vi "Motor_inlt.vi"(8 "에러 입력(에러 없음)":errorcluster) -> (0 "에러 출력":errorcluster)   [LabVIEW 2019]
uses:
  <vilib>/Platform/TimedLoop/XDataNode/timing_clust.ctl
  <vilib>/Platform/TimedLoop/XDataNode/nitl_modes.ctl
  <vilib>/Platform/TimedLoop/XDataNode/wakeup.ctl
  Type/SDO_Command.ctl
  <vilib>/Platform/TimedLoop/XDataNode/XDataNode.xnode
  <vilib>/Platform/TimedLoop/XDataNode/XDNodeRunTimeDep.lvlib
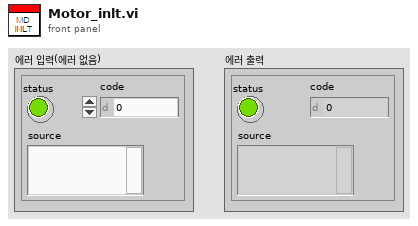
[diagram p1: front panel]
types:
  T1 = typedef "XDNodeRunTimeDep.lvlib/timing_clust.ctl" = cluster{"Expected End [f-1]":u64, "Actual End [f-1]":u64, "Finished Late? [f-1]":bool, "Expected End [i-1]":u64, "Actual End [i-1]":u64, "Finished Late? [i-1]":bool, "Expected Start [i]":u64, "Actual Start [i]":u64, "Expected Start [f]":u64, "Actual Start [f]":u64, "Source Name":string, "Structure Name":string, "Period":i64, "Deadline":i64, "Offset":i64, "Start":i64, "Priority":i32, "Timeout":i32, "Mode":T2, "Wakeup Reason":T3, "Error":errorcluster, "Source Type":string, "Secondary Source Type":string, "Global End Time":u64, "Global Start Time":u64, "Frame Duration":u64, "Iteration Duration":u64, "Assigned CPU":i32, "I/O Scan Engine Mode":u32}
  T2 = typedef "XDNodeRunTimeDep.lvlib/nitl_modes.ctl" = enum32{"No Change", "Process missed periods, maintain original phase", "Discard missed periods, maintain original phase", "Process missed periods, ignore original phase", "Discard missed periods, ignore original phase"}
  T3 = typedef "XDNodeRunTimeDep.lvlib/wakeup.ctl" = enum32{"Normal", "Aborted", "Asynchronous wakeup", "Timing source error", "Timed loop error", "Timeout"}
  T4 = cluster{"Target":i32, "Manual":u8[], "Velocity":u32, "Acc/Dec":u32}
  T5 = typedef "SDO_Command.ctl" = enum16{"Idle", "Shutdown", "Switch On", "Enable Operation", "Disable Voltage", "Quikstop", "Disable Operation", "Fault Reset", "Manual", "Statusword", "Mode of Operation", "Mode Display", "Target Position", "Position Actual Value", "Controlword_Move", "Profile Velocity", "Profile Acceleration", "Profile Deceleration", "Move"}
  T6 = typedef "CANFrameControl.ctl" = cluster{"identifier":u32, "extended?":bool, "type":u8, "payload":u8[]}
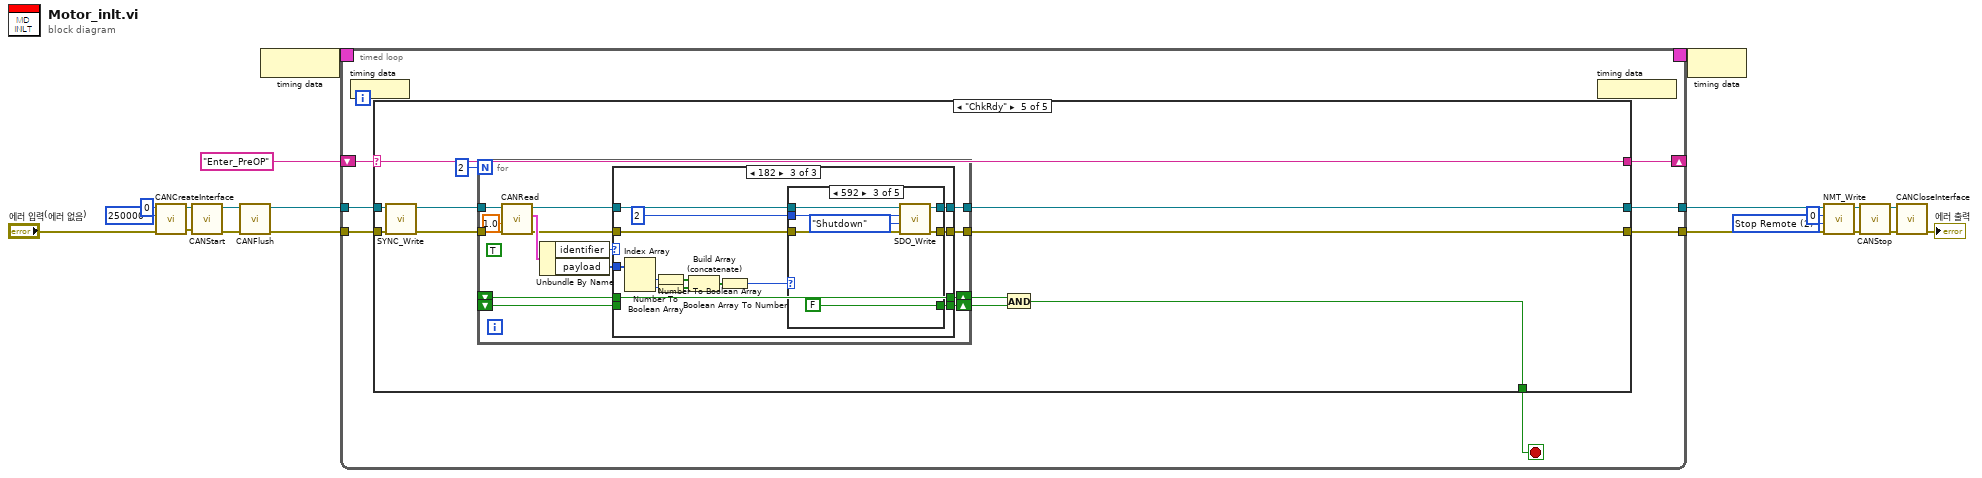
[diagram p0: block diagram]
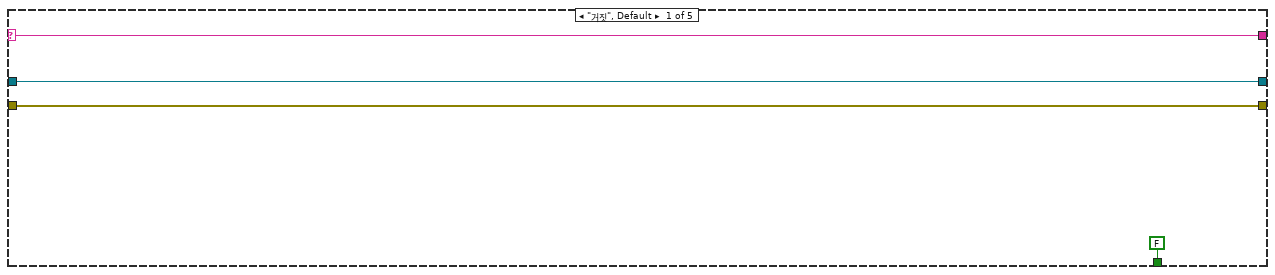
[diagram p2: hidden frame]
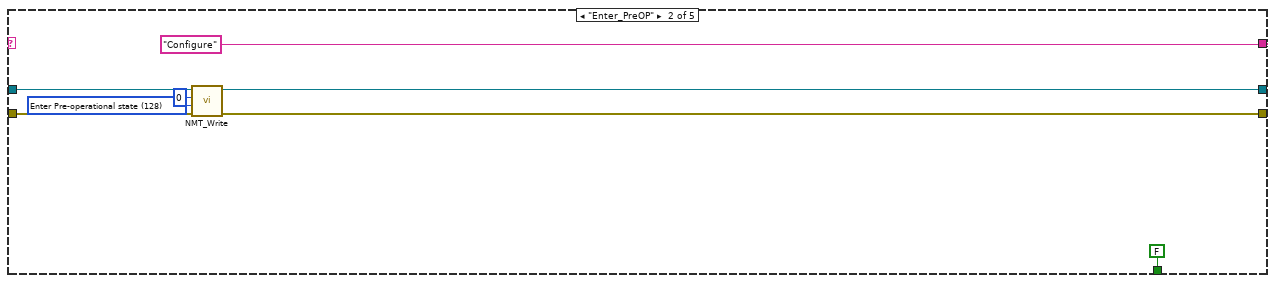
[diagram p3: hidden frame]
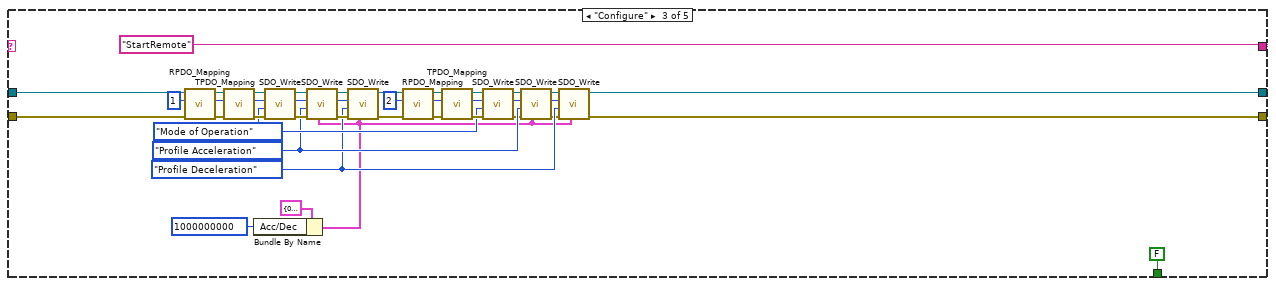
[diagram p4: hidden frame]
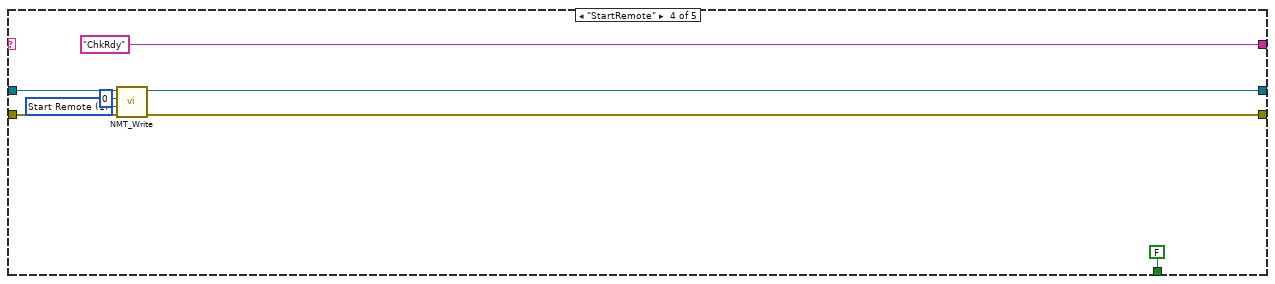
[diagram p5: hidden frame]
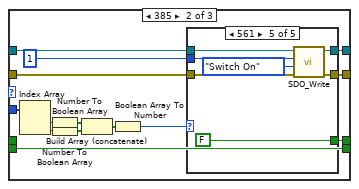
[diagram p7: hidden frame]
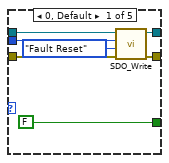
[diagram p8: hidden frame]
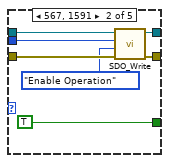
[diagram p9: hidden frame]
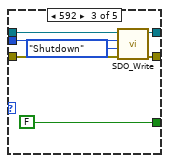
[diagram p10: hidden frame]
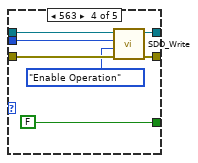
[diagram p11: hidden frame]
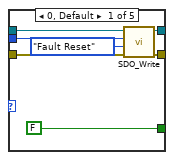
[diagram p12: hidden frame]
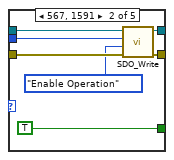
[diagram p13: hidden frame]
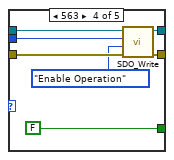
[diagram p14: hidden frame]
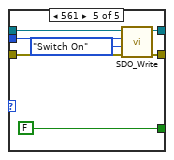
[diagram p15: hidden frame]
diagram:
  w15 = u8 2 items=["Start Remote"=1, "Stop Remote"=2, "Enter Pre-operational state"=128, "Reset node"=129, "Reset communication"=130] ("Command")
  n1 = call <vilib>:"CANCreateInterface.vi"("error in (no error)"="에러 입력(에러 없음)", "baud rate (125000 bps)"=u32 250000, "interface index"=u32 0) -> ("error out"=w4:errorcluster, "interface object out"=w3:refnum<k20>)  [unwired: 7 in]
  n2 = call <vilib>:"CANStart.vi"("error in (no error)"=w4, "interface object in"=w3) -> ("error out"=w7:errorcluster, "interface object out"=w6:refnum<k20>)  [unwired: 8 in]
  n3 = call <vilib>:"CANFlush.vi"("error in (no error)"=w7, "interface object in"=w6) -> ("error out"=w9:errorcluster, "interface object out"=w8:refnum<k20>)  [unwired: 8 in]
  n4 = node-c288() -> (w21:T1)
  n5 = timed-loop {
    shift-right: [w28] -> _
    shift-left: "Enter_PreOP" -> [w27]
    tunnel: [w26] -> w17
    timing: w21 -> [_]
    timing-out: [_] -> w20
    tunnel: w9 -> [w24]
    tunnel: w8 -> [w23]
    tunnel: [w25] -> w16
    stop <- w22 stop-if-true
    n6 = node-c288() -> ()  [unwired: 1 in]
    n7 = case shown="\"ChkRdy\"" w27 {
      selector: w27 -> [w34 _ _ _ w84]
      tunnel: [w34 "Configure" "StartRemote" "ChkRdy" w84] -> w28
      tunnel: [w33 w37 w45 w77 w89] -> w25
      tunnel: w23 -> [w33 w40 w48 w80 w91]
      tunnel: [w32 w36 w44 w76 w88] -> w26
      tunnel: w24 -> [w32 w39 w47 w79 w90]
      tunnel: [FALSE FALSE FALSE FALSE w83] -> w22
      frame "거짓", Default {
      }
      frame "Enter_PreOP" {
        w42 = u8 128 items=["Start Remote"=1, "Stop Remote"=2, "Enter Pre-operational state"=128, "Reset node"=129, "Reset communication"=130] ("Command")
        n8 = call "NMT_Write.vi"("error in"=w39, "Command"=w42, "Node_ID"=u32 0, "interface object in"=w40) -> ("error out"=w36:errorcluster, "interface object out"=w37:refnum<k20>)  [unwired: 6 in]
      }
      frame "Configure" {
        w52 = SDO_Command."Profile Deceleration" ("Command")
        w53 = SDO_Command."Profile Acceleration" ("Command")
        w54 = u32 2 ("Node_ID")
        w65 = u32 1 ("Node_ID")
        w57 = SDO_Command."Mode of Operation" ("Command")
        n9 = call "RPDO_Mapping.vi"("error in"=w47, "Node_ID"=w65, "interface object in"=w48) -> ("error out"=w73:errorcluster, "interface object out"=w74:refnum<k20>)  [unwired: 7 in]
        n10 = call "TPDO_Mapping.vi"("error in"=w73, "Node_ID"=w65, "interface object in"=w74) -> ("error out"=w71:errorcluster, "interface object out"=w72:refnum<k20>)  [unwired: 7 in]
        n11 = Bundle By Name(cluster=T4 {"Target"=0, "Manual"=[], "Velocity"=0, "Acc/Dec"=0} ("Parameter"), "Acc/Dec"=u32 1000000000) -> (w51:T4)
        n12 = call "SDO_Write.vi"("error in"=w71, "Command"=w57, "Node_ID"=w65, "interface object in"=w72) -> ("error out"=w64:errorcluster, "interface object out"=w63:refnum<k20>)  [unwired: 6 in]
        n13 = call "SDO_Write.vi"("Parameter"=w51, "error in"=w64, "Command"=w53, "Node_ID"=w65, "interface object in"=w63) -> ("error out"=w62:errorcluster, "interface object out"=w66:refnum<k20>)  [unwired: 5 in]
        n14 = call "SDO_Write.vi"("Parameter"=w51, "error in"=w62, "Command"=w52, "Node_ID"=w65, "interface object in"=w66) -> ("error out"=w58:errorcluster, "interface object out"=w59:refnum<k20>)  [unwired: 5 in]
        n15 = call "RPDO_Mapping.vi"("error in"=w58, "Node_ID"=w54, "interface object in"=w59) -> ("error out"=w69:errorcluster, "interface object out"=w70:refnum<k20>)  [unwired: 7 in]
        n16 = call "TPDO_Mapping.vi"("error in"=w69, "Node_ID"=w54, "interface object in"=w70) -> ("error out"=w67:errorcluster, "interface object out"=w68:refnum<k20>)  [unwired: 7 in]
        n17 = call "SDO_Write.vi"("error in"=w67, "Command"=w57, "Node_ID"=w54, "interface object in"=w68) -> ("error out"=w50:errorcluster, "interface object out"=w56:refnum<k20>)  [unwired: 6 in]
        n18 = call "SDO_Write.vi"("Parameter"=w51, "error in"=w50, "Command"=w53, "Node_ID"=w54, "interface object in"=w56) -> ("error out"=w49:errorcluster, "interface object out"=w55:refnum<k20>)  [unwired: 5 in]
        n19 = call "SDO_Write.vi"("Parameter"=w51, "error in"=w49, "Command"=w52, "Node_ID"=w54, "interface object in"=w55) -> ("error out"=w44:errorcluster, "interface object out"=w45:refnum<k20>)  [unwired: 5 in]
      }
      frame "StartRemote" {
        w81 = u8 1 items=["Start Remote"=1, "Stop Remote"=2, "Enter Pre-operational state"=128, "Reset node"=129, "Reset communication"=130] ("Command")
        n20 = call "NMT_Write.vi"("error in"=w79, "Command"=w81, "Node_ID"=u32 0, "interface object in"=w80) -> ("error out"=w76:errorcluster, "interface object out"=w77:refnum<k20>)  [unwired: 6 in]
      }
      frame "ChkRdy" {
        n21 = call "SYNC_Write.vi"("error in"=w90, "interface object in"=w91) -> ("error out"=w92:errorcluster, "interface object out"=w93:refnum<k20>)  [unwired: 8 in]
        n22 = for {
          N: 2 -> [_]
          tunnel: w93 -> [w102]
          tunnel: [w99] -> w89
          tunnel: w92 -> [w101]
          tunnel: [w98] -> w88
          shift-right: [w97] -> w87
          shift-left: _ -> [w95]
          shift-right: [w96] -> w86
          shift-left: _ -> [w94]
          (unwired) TRUE
          n23 = call <vilib>:"CANRead.vi"("error in (no error)"=w101, "timeout (0 s)"=1.0, "interface object in"=w102) -> ("error out"=w103:errorcluster, "CAN frame"=w107:T6, "interface object out"=w104:refnum<k20>)  [unwired: 5 in, 1 out]
          n24 = Unbundle By Name(w107) -> ("identifier"=w106:u32, "payload"=w105:u8[])
          n25 = case shown="182" w106 {
            tunnel: w105 -> [_ w120 w169]
            tunnel: w104 -> [w110 w119 w166]
            tunnel: w103 -> [w111 w118 w165]
            tunnel: [w111 w117 w167] -> w98
            tunnel: [w110 w116 w168] -> w99
            tunnel: [w109 w114 w161] -> w97
            tunnel: [w108 w112 w163] -> w96
            tunnel: w95 -> [w109 _ w161]
            tunnel: w94 -> [w108 w112 _]
            frame 0, Default {
            }
            frame 385 {
              n26 = Index Array(array=w120) -> (element #1=w125:u8, element #2=w124:u8)  [unwired: 2 in]
              n27 = Number To Boolean Array(number=w125) -> (Boolean array=w123:bool[])
              n28 = Number To Boolean Array(number=w124) -> (Boolean array=w122:bool[])
              n29 = Build Array (concatenate)(w123, w122) -> (w121:bool[])
              n30 = Boolean Array To Number(Boolean array=w121) -> (number=w115:u32)
              n31 = case shown="561" w115 {
                tunnel: u32 1 -> [w130 w137 w144 w151 w158]
                tunnel: w119 -> [w131 w138 w145 w150 w159]
                tunnel: w118 -> [w129 w136 w143 w152 w157]
                tunnel: [FALSE TRUE FALSE FALSE FALSE] -> w114
                tunnel: [w127 w135 w141 w149 w156] -> w116
                tunnel: [w128 w134 w142 w148 w155] -> w117
                frame 0, Default {
                  n32 = call "SDO_Write.vi"("error in"=w129, "Command"=SDO_Command."Fault Reset", "Node_ID"=w130, "interface object in"=w131) -> ("error out"=w128:errorcluster, "interface object out"=w127:refnum<k20>)  [unwired: 6 in]
                }
                frame 567, 1591 {
                  n33 = call "SDO_Write.vi"("error in"=w136, "Command"=SDO_Command."Enable Operation", "Node_ID"=w137, "interface object in"=w138) -> ("error out"=w134:errorcluster, "interface object out"=w135:refnum<k20>)  [unwired: 6 in]
                }
                frame 592 {
                  n34 = call "SDO_Write.vi"("error in"=w143, "Command"=SDO_Command."Shutdown", "Node_ID"=w144, "interface object in"=w145) -> ("error out"=w142:errorcluster, "interface object out"=w141:refnum<k20>)  [unwired: 6 in]
                }
                frame 563 {
                  n35 = call "SDO_Write.vi"("error in"=w152, "Command"=SDO_Command."Enable Operation", "Node_ID"=w151, "interface object in"=w150) -> ("error out"=w148:errorcluster, "interface object out"=w149:refnum<k20>)  [unwired: 6 in]
                }
                frame 561 {
                  n36 = call "SDO_Write.vi"("error in"=w157, "Command"=SDO_Command."Switch On", "Node_ID"=w158, "interface object in"=w159) -> ("error out"=w155:errorcluster, "interface object out"=w156:refnum<k20>)  [unwired: 6 in]
                }
              }
            }
            frame 386 {
              n37 = Index Array(array=w169) -> (element #1=w174:u8, element #2=w173:u8)  [unwired: 2 in]
              n38 = Number To Boolean Array(number=w174) -> (Boolean array=w172:bool[])
              n39 = Number To Boolean Array(number=w173) -> (Boolean array=w171:bool[])
              n40 = Build Array (concatenate)(w172, w171) -> (w170:bool[])
              n41 = Boolean Array To Number(Boolean array=w170) -> (number=w164:u32)
              n42 = case shown="592" w164 {
                tunnel: u32 2 -> [w179 w185 w193 w200 w207]
                tunnel: w166 -> [w180 w186 w194 w201 w208]
                tunnel: w165 -> [w178 w187 w192 w199 w206]
                tunnel: [FALSE TRUE FALSE FALSE FALSE] -> w163
                tunnel: [w177 w184 w191 w198 w205] -> w168
                tunnel: [w176 w183 w190 w197 w204] -> w167
                frame 0, Default {
                  n43 = call "SDO_Write.vi"("error in"=w178, "Command"=SDO_Command."Fault Reset", "Node_ID"=w179, "interface object in"=w180) -> ("error out"=w176:errorcluster, "interface object out"=w177:refnum<k20>)  [unwired: 6 in]
                }
                frame 567, 1591 {
                  n44 = call "SDO_Write.vi"("error in"=w187, "Command"=SDO_Command."Enable Operation", "Node_ID"=w185, "interface object in"=w186) -> ("error out"=w183:errorcluster, "interface object out"=w184:refnum<k20>)  [unwired: 6 in]
                }
                frame 592 {
                  n45 = call "SDO_Write.vi"("error in"=w192, "Command"=SDO_Command."Shutdown", "Node_ID"=w193, "interface object in"=w194) -> ("error out"=w190:errorcluster, "interface object out"=w191:refnum<k20>)  [unwired: 6 in]
                }
                frame 563 {
                  n46 = call "SDO_Write.vi"("error in"=w199, "Command"=SDO_Command."Enable Operation", "Node_ID"=w200, "interface object in"=w201) -> ("error out"=w197:errorcluster, "interface object out"=w198:refnum<k20>)  [unwired: 6 in]
                }
                frame 561 {
                  n47 = call "SDO_Write.vi"("error in"=w206, "Command"=SDO_Command."Switch On", "Node_ID"=w207, "interface object in"=w208) -> ("error out"=w204:errorcluster, "interface object out"=w205:refnum<k20>)  [unwired: 6 in]
                }
              }
            }
          }
        }
        n48 = And(x=w87, y=w86) -> (x .and. y?=w83:bool)
      }
    }
    n49 = node-c288() -> ()  [unwired: 1 out]
  }
  n50 = node-c288(w20) -> ()
  n51 = call "NMT_Write.vi"("error in"=w17, "Command"=w15, "Node_ID"=u32 0, "interface object in"=w16) -> ("error out"=w13:errorcluster, "interface object out"=w12:refnum<k20>)  [unwired: 6 in]
  n52 = call <vilib>:"CANStop.vi"("error in (no error)"=w13, "interface object in"=w12) -> ("error out"=w10:errorcluster, "interface object out"=w11:refnum<k20>)  [unwired: 8 in]
  n53 = call <vilib>:"CANCloseInterface.vi"("error in (no error)"=w10, "interface object in"=w11) -> ("error out"=→"에러 출력":errorcluster)  [unwired: 9 in]
